vi "Lock Focus Knob.vi"(0 "Notifier Name In":string, 7 "Lock Focus Knob":bool, 11 "Error In":errorcluster) -> (4 "Notifier Name Out":string, 15 "Error Out":errorcluster)   [LabVIEW 2020]
uses:
  Microscopes Type Defs/Microscope Notifier.ctl
  Microscopes Type Defs/Microscope Actions.ctl
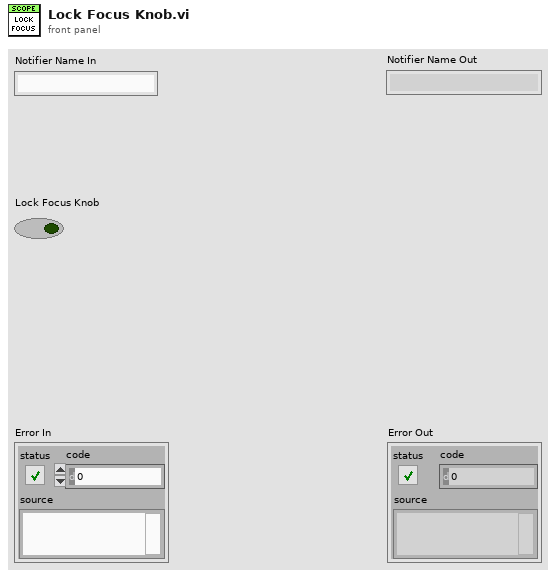
[diagram p1: front panel]
types:
  T1 = typedef "Microscope Notifier.ctl" = cluster{"Actions":T2, "Action Done":bool, "Objective Index":u8, "Objective Z Position (um)":dbl, "Lamp Index":u8, "Lamp State":bool, "Output Port":u8, "Shutter Index":u8, "Shutter State":bool, "Dichroic Wheel Position":u8, "Parameter":string, "Parameter Value":string, "Base Locked?":bool, "Obj Speed":u32, "Obj Acceleration":u32, "Obj Deceleration":u32, "Lamp Power (%)":dbl, "Dichroic Wheel Index":u8}
  T2 = typedef "Microscope Actions.ctl" = enum16{"Do Nothing", "Lock Base", "Lock Focus Knob", "Get Objective Index", "Get Objective Z Position", "Get Lamp State", "Get Lamp Power", "Get Output Port", "Get Shutter State", "Get Dichroic Wheel Position", "Set Lamp Index", "Set Shutter Index", "Set Objective Z Position", "Set Lamp State", "Set Lamp Power", "Set Output Port", "Set Shutter State", "Set Dichroic Wheel Position", "Set Objective", "Abort Move", "Set Parameter", "Get Parameter", "Quit"}
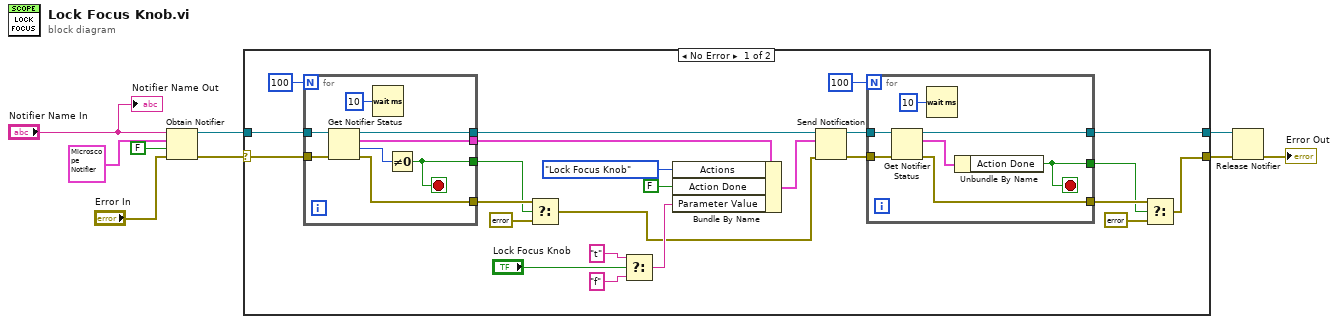
[diagram p0: block diagram]
diagram:
  n1 = Obtain Notifier(name (unnamed)="Notifier Name In", notification data type=T1 {"Actions"=enum."Get Objective Index", "Action Done"=FALSE, "Objective Index"=0, "Objective Z Position (um)"=0.0, "Lamp Index"=0, "Lamp State"=FALSE, "Output Port"=0, "Shutter Index"=0, "Shutter State"=FALSE, "Dichroic Wheel Position"=0, "Parameter"="", "Parameter Value"="", "Base Locked?"=FALSE, "Obj Speed"=0, "Obj Acceleration"=0, "Obj Deceleration"=0, "Lamp Power (%)"=0.0, "Dichroic Wheel Index"=0} ("Microscope Notifier"), create if not found? (T)=FALSE, error in (no error)="Error In") -> (notifier out=w6:refnum<notifier>, error out=w7:errorcluster)  [unwired: 1 out]
  n2 = case shown="No Error" w7 {
    selector: w7 -> [w31 w50]
    tunnel: w6 -> [w33 w49]
    tunnel: [w22 w50] -> w2
    tunnel: [w23 w49] -> w3
    frame No Error {
      n3 = for {
        N: 100 -> [_]
        tunnel: w33 -> [w48]
        tunnel: [w46] -> w19
        tunnel: [w44] -> w29
        tunnel: w31 -> [w43]
        tunnel: [w42] -> w20
        tunnel: [w41] -> w30
        stop <- w46 stop-if-true
        n4 = Get Notifier Status(notifier=w48, error in (no error)=w43) -> (notifier out=w44:refnum<notifier>, current notification=w41:T1, # waiting=w47:i32, error out=w42:errorcluster)  [unwired: 1 out]
        n5 = Wait (ms)(milliseconds to wait=u32 10) -> ()  [unwired: 1 out]
        n6 = Not Equal To 0?(x=w47) -> (x != 0?=w46:bool)
      }
      n7 = Select(t=w20, s=w19, f=errorcluster {"status"=TRUE, "code"=0, "source"="IX81 Base Error: Base busy time out."}) -> (s? t:f=w10:errorcluster)
      n8 = Select(t="t", s="Lock Focus Knob", f="f") -> (s? t:f=w15:string)
      n9 = Bundle By Name(cluster=w30, "Actions"=Microscope_Actions."Lock Focus Knob", "Action Done"=FALSE, "Parameter Value"=w15) -> (w28:T1)
      n10 = Send Notification(notification=w28, notifier=w29, error in (no error)=w10) -> (notifier out=w24:refnum<notifier>, error out=w27:errorcluster)
      n11 = for {
        N: 100 -> [_]
        tunnel: w24 -> [w40]
        tunnel: [w38] -> w23
        tunnel: w27 -> [w37]
        tunnel: [w36] -> w13
        tunnel: [w34] -> w12
        stop <- w34 stop-if-true
        n12 = Get Notifier Status(notifier=w40, error in (no error)=w37) -> (notifier out=w38:refnum<notifier>, current notification=w35:T1, error out=w36:errorcluster)  [unwired: 2 out]
        n13 = Wait (ms)(milliseconds to wait=u32 10) -> ()  [unwired: 1 out]
        n14 = Unbundle By Name(w35) -> ("Action Done"=w34:bool)
      }
      n15 = Select(t=w13, s=w12, f=errorcluster {"status"=TRUE, "code"=0, "source"="IX81 Base Error: Action didn't complete."}) -> (s? t:f=w22:errorcluster)
    }
    frame Error {
    }
  }
  n16 = Release Notifier(notifier=w3, error in (no error)=w2) -> (error out=→"Error Out":errorcluster)  [unwired: 1 in, 2 out]
  "Notifier Name Out" <- "Notifier Name In"
